vi "Find.vi"(8 "Error In":errorcluster, 10 "Key":string, 11 "Context In":refnum<class "Context.lvclass">) -> (0 "Error Out":errorcluster, 1 "Found?":bool, 2 "Datum":refnum<class "Datum.lvclass">, 3 "Context Out":refnum<class "Context.lvclass">)   [LabVIEW 2018, in "Toolkit.lvlib" / "Context.lvclass"]
doc: "Finds a value associated with the key within the context."
uses:
  Context.lvclass
  Data/Datum/Datum.lvclass
  Context.lvclass/Context.ctl
  Data/Null/Null.lvclass
  D:/Users/cfield/Code/Field R&D Services/Labstache/src/Toolkit/Data/Datum/Datum.lvclass
  Data/Map/Map.lvclass
  Data/Pair/Pair.lvclass
  Data/Pair/Pair.lvclass/Pair.ctl
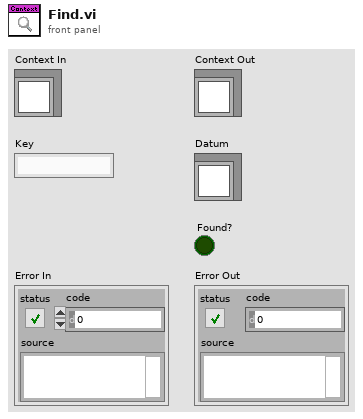
[diagram p1: front panel]
types:
  T1 = typedef "Toolkit.lvlib/Data.lvlib/Types.ctl" = enum16{"Array", "Boolean", "Function", "Map", "Null", "Pair", "Path", "String", "Unknown"}
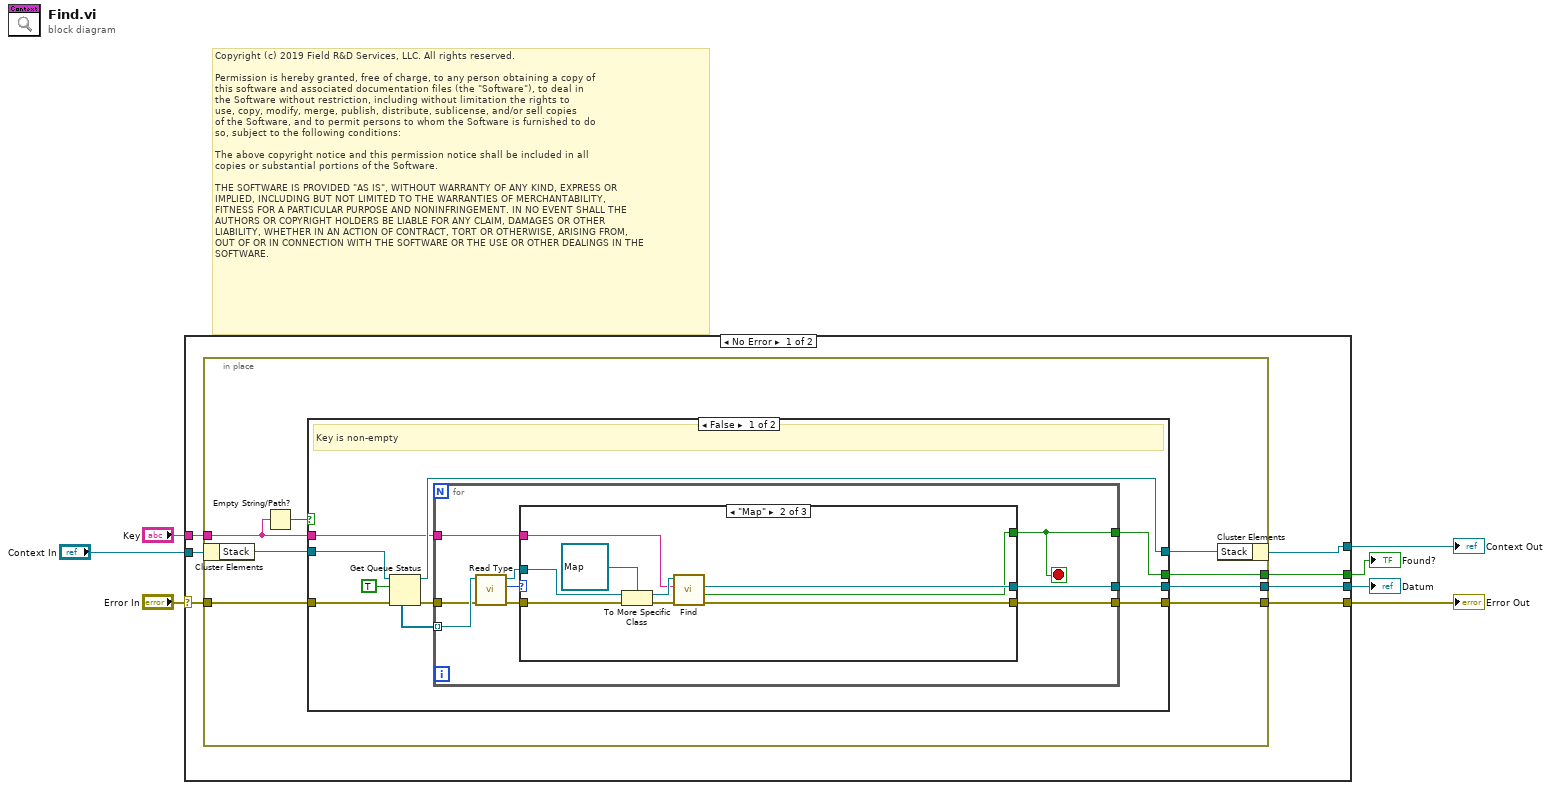
[diagram p0: block diagram]
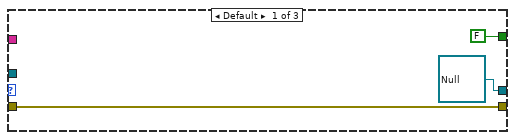
[diagram p2: hidden frame]
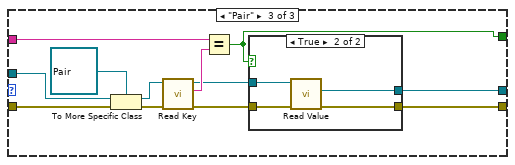
[diagram p3: hidden frame]
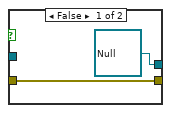
[diagram p4: hidden frame]
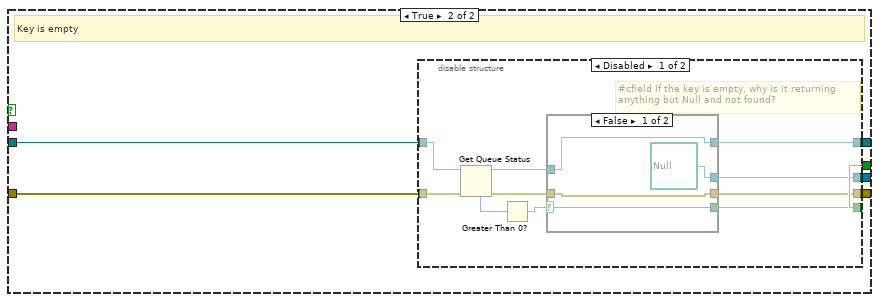
[diagram p5: hidden frame]
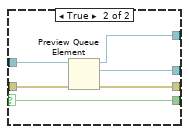
[diagram p6: hidden frame]
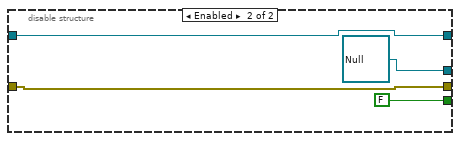
[diagram p7: hidden frame]
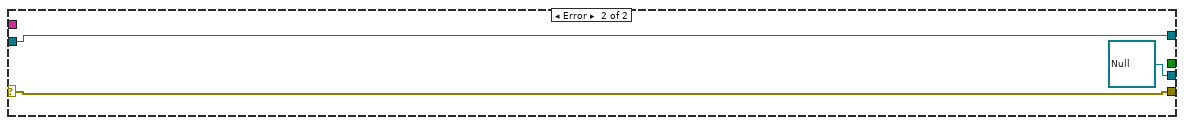
[diagram p8: hidden frame]
diagram:
  # "Copyright (c) 2019 Field R&D Services, LLC. All rights reserved.\n\nPermission is hereby granted, free of charge, to any person obtaining a copy of\nthis software and associated documentation files (the \"Software\"), to deal in\nthe Software without restriction, including without limitation the rights to\nuse, copy, modify, merge, publish, distribute, sublicense, and/or sell copies\nof the Software, and to permit persons to whom the Software is furnished to do\nso, subject to the following conditions:\n\nThe above copyright notice and this permission notice shall be included in all\ncopies or substantial portions of the Software.\n\nTHE SOFTWARE IS PROVIDED \"AS IS\", WITHOUT WARRANTY OF ANY KIND, EXPRESS OR\nIMPLIED, INCLUDING BUT NOT LIMITED TO THE WARRANTIES OF MERCHANTABILITY,\nFITNESS FOR A PARTICULAR PURPOSE AND NONINFRINGEMENT. IN NO EVENT SHALL THE\nAUTHORS OR COPYRIGHT HOLDERS BE LIABLE FOR ANY CLAIM, DAMAGES OR OTHER\nLIABILITY, WHETHER IN AN ACTION OF CONTRACT, TORT OR OTHERWISE, ARISING FROM,\nOUT OF OR IN CONNECTION WITH THE SOFTWARE OR THE USE OR OTHER DEALINGS IN THE\nSOFTWARE."
  n1 = case shown="No Error" "Error In" {
    selector: "Error In" -> [w11 w103]
    tunnel: [w14 refnum<class "Null.lvclass"> refnum ("Toolkit.lvlib:Data.lvlib:Null.lvclass")] -> w7
    tunnel: [w13 w103] -> w6
    tunnel: [w12 _] -> w5
    tunnel: "Context In" -> [w10 w104]
    tunnel: [w9 w104] -> w2
    tunnel: "Key" -> [w8 _]
    frame No Error {
      n2 = in-place {
        in-place-border: [w22] -> w14
        in-place-border: [w21] -> w13
        in-place-border: [w20] -> w12
        in-place-border: w11 -> [w19]
        in-place-border: w8 -> [w16]
        n3 = in-place-cluster #1(w10) -> ("Stack"=w18:refnum<queue>)
        n4 = Empty String/Path?(string/path=w16) -> (empty?=w15:bool)
        n5 = case shown="False" w15 {
          tunnel: [w32 w76] -> w22
          tunnel: [w31 w72] -> w21
          tunnel: [w27 w73] -> w20
          tunnel: w19 -> [w26 w74]
          tunnel: w18 -> [w25 w75]
          tunnel: [w24 w77] -> w17
          tunnel: w16 -> [w23 _]
          frame False {
            # "Key is non-empty"
            n6 = Get Queue Status(queue=w25, return elements? (F)=TRUE, error in (no error)=w26) -> (queue out=w24:refnum<queue>, error out=w30:errorcluster, elements=w29:refnum<class "Datum.lvclass">[])  [unwired: 5 out]
            n7 = for {
              tunnel: w29 -> [w37] mode=indexing
              tunnel: w23 -> [w41]
              tunnel: w30 -> [w35]
              tunnel: [w40] -> w31
              tunnel: [w39] -> w32
              tunnel: [w38] -> w27
              stop <- w38 stop-if-true
              n8 = call-dynamic "Read Type.vi"("Error In"=w35, "Datum In"=w37) -> ("Error Out"=w34:errorcluster, "Type"=w33:T1, "Datum Out"=w36:refnum<class "Datum.lvclass">)  [unwired: 7 in]
              n9 = case shown="\"Map\"" w33 {
                tunnel: w34 -> [w43 w53 w65]
                tunnel: w36 -> [_ w52 w64]
                tunnel: w41 -> [_ w48 w59]
                tunnel: [w43 w47 w56] -> w40
                tunnel: [FALSE ("Found?") w45 w58] -> w38
                tunnel: [refnum<class "Null.lvclass"> refnum ("Toolkit.lvlib:Data.lvlib:Null.lvclass") w46 w54] -> w39
                frame Default {
                }
                frame "Map" {
                  n10 = To More Specific Class(target class=refnum<class "Map.lvclass"> refnum ("Toolkit.lvlib:Data.lvlib:Map.lvclass"), reference=w52, error in=w53) -> (specific class reference=w49:refnum<class "Map.lvclass">, error out=w50:errorcluster)
                  n11 = call "Find.vi"("Error In"=w50, "Key"=w48, "Map In"=w49) -> ("Error Out"=w47:errorcluster, "Found?"=w45:bool, "Value"=w46:refnum<class "Datum.lvclass">)  [unwired: 5 in, 1 out]
                }
                frame "Pair" {
                  n12 = To More Specific Class(target class=refnum<class "Pair.lvclass"> refnum ("Toolkit.lvlib:Data.lvlib:Pair.lvclass"), reference=w64, error in=w65) -> (specific class reference=w62:refnum<class "Pair.lvclass">, error out=w61:errorcluster)
                  n13 = call "Read Key.vi"("Error In"=w61, "Pair In"=w62) -> ("Error Out"=w57:errorcluster, "Key"=w60:string, "Pair Out"=w55:refnum<class "Pair.lvclass">)  [unwired: 7 in]
                  n14 = Equal?(x=w59, y=w60) -> (x = y?=w58:bool)
                  n15 = case shown="True" w58 {
                    tunnel: w57 -> [w67 w71]
                    tunnel: [w67 w70] -> w56
                    tunnel: w55 -> [_ w69]
                    tunnel: [refnum<class "Null.lvclass"> refnum ("Toolkit.lvlib:Data.lvlib:Null.lvclass") w68] -> w54
                    frame False {
                    }
                    frame True {
                      n16 = call "Read Value.vi"("Error In"=w71, "Pair In"=w69) -> ("Error Out"=w70:errorcluster, "Value"=w68:refnum<class "Datum.lvclass">)  [unwired: 7 in, 1 out]
                    }
                  }
                }
              }
            }
          }
          frame True {
            # "Key is empty"
            n17 = disable-structure "Diagram Disable Structure" shown="Disabled" {
              disable-tunnel: [w87 w101] -> w77
              disable-tunnel: [w86 refnum<class "Null.lvclass"> refnum ("Toolkit.lvlib:Data.lvlib:Null.lvclass")] -> w76
              disable-tunnel: w75 -> [w85 w101]
              disable-tunnel: w74 -> [w82 w100]
              disable-tunnel: [w79 FALSE] -> w73
              disable-tunnel: [w78 w100] -> w72
              frame Disabled {
                # "#cfield If the key is empty, why is it returning anything but Null and not found?"
                n18 = Get Queue Status(queue=w85, error in (no error)=w82) -> (queue out=w84:refnum<queue>, error out=w83:errorcluster, # elements in queue=w81:i32)  [unwired: 1 in, 5 out]
                n19 = Greater Than 0?(x=w81) -> (x > 0?=w80:bool)
                n20 = case shown="False" w80 {
                  selector: w80 -> [w90 w92]
                  tunnel: [w91 w97] -> w87
                  tunnel: [refnum<class "Null.lvclass"> refnum ("Toolkit.lvlib:Data.lvlib:Null.lvclass") w96] -> w86
                  tunnel: w84 -> [w91 w95]
                  tunnel: w83 -> [w89 w94]
                  tunnel: [w90 w92] -> w79
                  tunnel: [w89 w93] -> w78
                  frame False {
                  }
                  frame True {
                    n21 = Preview Queue Element(queue=w95, error in (no error)=w94) -> (queue out=w97:refnum<queue>, element=w96:refnum<class "Datum.lvclass">, error out=w93:errorcluster)  [unwired: 1 in, 1 out]
                  }
                }
              }
              frame Enabled {
              }
            }
          }
        }
        n22 = in-place-cluster #1("Stack"=w17) -> (w9:refnum<class "Context.lvclass">)
      }
    }
    frame Error {
    }
  }
  "Datum" <- w7
  "Error Out" <- w6
  "Found?" <- w5
  "Context Out" <- w2
